vi "onDisconnection.vi"(8 "error in (no error)":errorcluster, 11 "Connection":refnum<class "Connection.lvclass">) -> (0 "error out":errorcluster, 3 "No connection":refnum<class "Connection.lvclass">)   [LabVIEW 2013, in "Connection_GOSPL.lvlib" / "Connection.lvclass"]
uses:
  Connection.lvclass
  Connection.lvclass/Connection.ctl
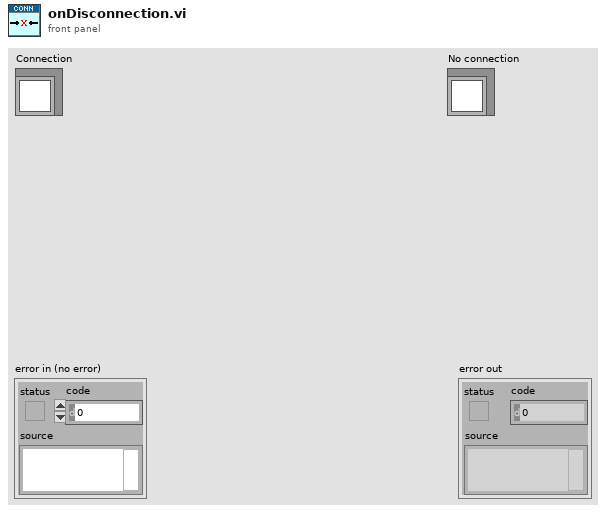
[diagram p1: front panel]
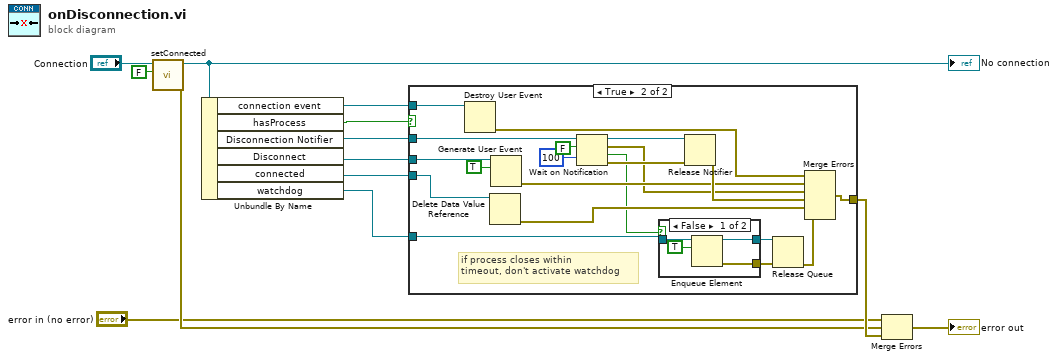
[diagram p0: block diagram]
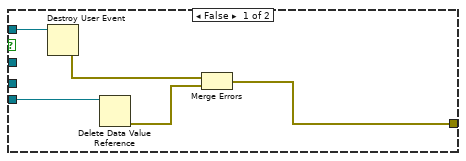
[diagram p2: hidden frame]
diagram:
  n1 = call "setConnected.vi"("connected"=FALSE, "Connection in"="Connection") -> ("error out"=w3:errorcluster, "Connection out"=w4:refnum<class "Connection.lvclass">)  [unwired: 8 in]
  "No connection" <- w4
  n2 = Unbundle By Name(w4) -> ("connection event"=w2:refnum<user-event>, "hasProcess"=w9:bool, "Disconnection Notifier"=w12:refnum<notifier>, "Disconnect"=w13:refnum<user-event>, "connected"=w8:refnum<data-value>, "watchdog"=w7:refnum<queue>)
  n3 = case shown="True" w9 {
    tunnel: w13 -> [_ w38]
    tunnel: w12 -> [_ w37]
    tunnel: [w14 w30] -> w11
    tunnel: w8 -> [w18 w29]
    tunnel: w7 -> [_ w25]
    tunnel: w2 -> [w17 w20]
    frame False {
      n4 = Destroy User Event(user event=w17) -> (error out=w16:errorcluster)  [unwired: 1 in]
      n5 = Delete Data Value Reference(data value reference=w18) -> (error out=w15:errorcluster)  [unwired: 1 in, 1 out]
      n6 = Merge Errors(w16, w15) -> (w14:errorcluster)
    }
    frame True {
      # "if process closes within\ntimeout, don't activate watchdog"
      n7 = Destroy User Event(user event=w20) -> (error out=w19:errorcluster)  [unwired: 1 in]
      n8 = Delete Data Value Reference(data value reference=w29) -> (error out=w28:errorcluster)  [unwired: 1 in, 1 out]
      n9 = Generate User Event(user event=w38, event data cluster=TRUE ("event data")) -> (error out=w31:errorcluster)  [unwired: 2 in, 1 out]
      n10 = Wait on Notification(notifier=w37, ignore previous (F)=FALSE, timeout in ms (-1)=100) -> (notifier out=w33:refnum<notifier>, notification=w26:errorcluster, timed out?=w21:bool, error out=w27:errorcluster)  [unwired: 1 in]
      n11 = case shown="False" w21 {
        tunnel: w25 -> [w42 w43]
        tunnel: [w41 w43] -> w24
        tunnel: [w39 _] -> w23
        frame False {
          n12 = Enqueue Element(queue=w42, element=TRUE) -> (queue out=w41:refnum<queue>, error out=w39:errorcluster)  [unwired: 2 in, 1 out]
        }
        frame True {
        }
      }
      n13 = Release Notifier(notifier=w33, error in (no error)=w27) -> (error out=w32:errorcluster)  [unwired: 1 in, 2 out]
      n14 = Release Queue(queue=w24, error in (no error)=w23) -> (error out=w22:errorcluster)  [unwired: 1 in, 2 out]
      n15 = Merge Errors(w19, w31, w26, w32, w28, w22) -> (w30:errorcluster)
    }
  }
  n16 = Merge Errors("error in (no error)", w3, w11) -> (→"error out":errorcluster)
